vi "Generate Pulse Train Testing.vi"(11 "O3 Frequency Train Actor in":refnum<class "O3 Frequency Train Actor.lvclass">) -> ()   [LabVIEW 2014, in "Calibration.lvlib" / "O3 Frequency Train Actor.lvclass"]
uses:
  O3 Frequency Train Actor.lvclass
  <vilib>/Platform/TimedLoop/XDataNode/nitl_modes.ctl
  <vilib>/Platform/TimedLoop/XDataNode/timing_clust.ctl
  <vilib>/Platform/TimedLoop/XDataNode/wakeup.ctl
  O3 Frequency Train Actor.lvclass/O3 Frequency Train Actor.ctl
  <vilib>/DAQmx/write.llb/DAQmx Write (Digital Bool 1Line 1Point).vi
  <vilib>/Platform/TimedLoop/XDataNode/XDataNode.xnode
  <vilib>/Platform/TimedLoop/XDataNode/XDNodeRunTimeDep.lvlib
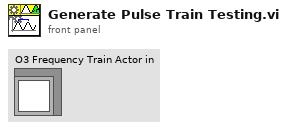
[diagram p1: front panel]
types:
  T1 = typedef "XDNodeRunTimeDep.lvlib/nitl_modes.ctl" = enum32{"No Change", "Process missed periods, maintain original phase", "Discard missed periods, maintain original phase", "Process missed periods, ignore original phase", "Discard missed periods, ignore original phase"}
  T2 = typedef "XDNodeRunTimeDep.lvlib/timing_clust.ctl" = cluster{"Expected End [f-1]":u64, "Actual End [f-1]":u64, "Finished Late? [f-1]":bool, "Expected End [i-1]":u64, "Actual End [i-1]":u64, "Finished Late? [i-1]":bool, "Expected Start [i]":u64, "Actual Start [i]":u64, "Expected Start [f]":u64, "Actual Start [f]":u64, "Source Name":string, "Structure Name":string, "Period":i64, "Deadline":i64, "Offset":i64, "Start":i64, "Priority":i32, "Timeout":i32, "Mode":T1, "Wakeup Reason":T3, "Error":errorcluster, "Source Type":string, "Secondary Source Type":string, "Global End Time":u64, "Global Start Time":u64, "Frame Duration":u64, "Iteration Duration":u64, "Assigned CPU":i32, "I/O Scan Engine Mode":u32}
  T3 = typedef "XDNodeRunTimeDep.lvlib/wakeup.ctl" = enum32{"Normal", "Aborted", "Asynchronous wakeup", "Timing source error", "Timed loop error", "Timeout"}
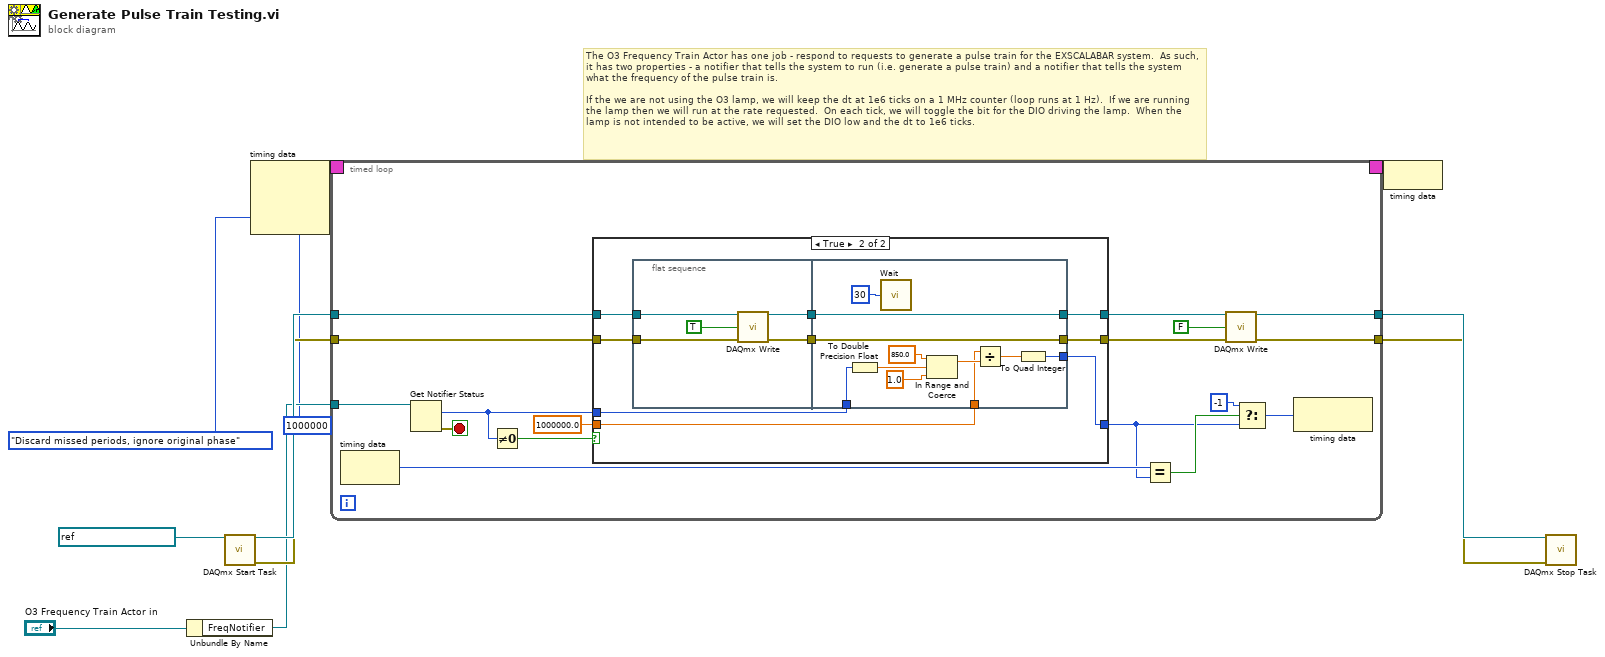
[diagram p0: block diagram]
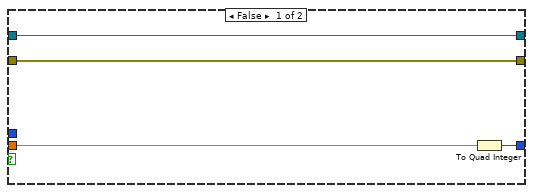
[diagram p2: hidden frame]
diagram:
  # "The O3 Frequency Train Actor has one job - respond to requests to generate a pulse train for the EXSCALABAR system.  As such, it has two properties - a notifier that tells the system to run (i.e. generate a pulse train) and a notifier that tells the system what the frequency of the pulse train is.  \n\nIf the we are not using the O3 lamp, we will keep the dt at 1e6 ticks on a 1 MHz counter (loop runs at 1 Hz).  If we are running the lamp then we will run at the rate requested.  On each tick, we will toggle the bit for the DIO driving the lamp.  When the lamp is not intended to be active, we will set the DIO low and the dt to 1e6 ticks."
  n1 = Unbundle By Name("O3 Frequency Train Actor in") -> ("FreqNotifier"=w5:refnum<notifier>)
  n2 = call <vilib>:"DAQmx Start Task.vi"("task/channels in"=refnum<k21> "O3 Lamp Output") -> ("task out"=w8:refnum<k21>, "error out"=w7:errorcluster)  [unwired: 13 in]
  n3 = node-c288(i64 1000000 ("Period"), nitl_modes."Discard missed periods, ignore original phase" ("Mode")) -> (w11:T2)  [unwired: 1 in]
  n4 = timed-loop {
    timing: w11 -> [_]
    timing-out: [_] -> w10
    tunnel: w8 -> [w28]
    tunnel: [w19] -> w9
    tunnel: w7 -> [w27]
    tunnel: [w18] -> w6
    tunnel: w5 -> [w26]
    stop <- w20 stop-if-true
    n5 = node-c288() -> (w23:i64)  [unwired: 1 in]
    n6 = Get Notifier Status(notifier=w26) -> (current notification=w12:i64, error out=w20:errorcluster)  [unwired: 1 in, 3 out]
    n7 = Not Equal To 0?(x=w12) -> (x != 0?=w15:bool)
    n8 = case shown="True" w15 {
      tunnel: w28 -> [w32 w41]
      tunnel: w27 -> [w31 w40]
      tunnel: [w31 w39] -> w16
      tunnel: [w32 w38] -> w17
      tunnel: [w29 w35] -> w21
      tunnel: 1000000.0 ("x") -> [w30 w34]
      tunnel: w12 -> [_ w33]
      frame False {
        n9 = To Quad Integer(1:w30) -> (0:w29:i64)
      }
      frame True {
        n10 = flat-sequence {
          tunnel: w41 -> [w46]
          tunnel: w40 -> [w45]
          tunnel: [w44] -> w37
          tunnel: [w43] -> w36
          tunnel: [w56] -> w38
          tunnel: [w57] -> w39
          tunnel: w37 -> [w57]
          tunnel: w36 -> [w56]
          tunnel: [w50] -> w35
          tunnel: w34 -> [w49]
          tunnel: w33 -> [w47]
          frame #0 {
            n11 = call-poly <vilib>:"DAQmx Write.vi"("task/channels in"=w46, "data"=TRUE ("auto start"), "error in"=w45) -> ("task out"=w43:refnum<k21>, "error out"=w44:errorcluster)  [unwired: 10 in, 1 out]
          }
          frame #1 {
            n12 = To Double Precision Float(number=w47) -> (double precision float=w48:dbl)
            n13 = call "Wait"("Count(uSec)"=u32 30) -> ()  [unwired: 1 out]
            n14 = In Range and Coerce(upper limit=850.0, x=w48, lower limit=1.0) -> (coerced(x)=w54:dbl)  [unwired: 1 out]
            n15 = Divide(x=w49, y=w54) -> (x/y=w52:dbl)
            n16 = To Quad Integer(1:w52) -> (0:w50:i64)
          }
        }
      }
    }
    n17 = Equal?(x=w23, y=w21) -> (x = y?=w24:bool)
    n18 = call-poly <vilib>:"DAQmx Write.vi"("task/channels in"=w17, "data"=FALSE, "error in"=w16) -> ("task out"=w19:refnum<k21>, "error out"=w18:errorcluster)  [unwired: 10 in, 1 out]
    n19 = Select(t=i64 -1, s=w24, f=w21) -> (s? t:f=w22:i64)
    n20 = node-c288(w22) -> ()  [unwired: 1 out]
  }
  n21 = node-c288(w10) -> ()
  n22 = call <vilib>:"DAQmx Stop Task.vi"("task/channels in"=w9, "error in"=w6) -> ()  [unwired: 12 in, 2 out]
